vi "WriteExcel.vi"(8 "error in (no error)":errorcluster caption="错误输入（无错误）", 10 "Data":string[][](array[string]), 11 "Path":path=path "C:/Users/ct/Desktop/TestStep.xlsx") -> (0 "error out":errorcluster caption="错误输出")   [LabVIEW 2017]
uses:
  <vilib>/Utility/NIReport.llb/NI_report.lvclass
  <vilib>/Utility/NIReport.llb/Append Text Table to Report (wrap).vi
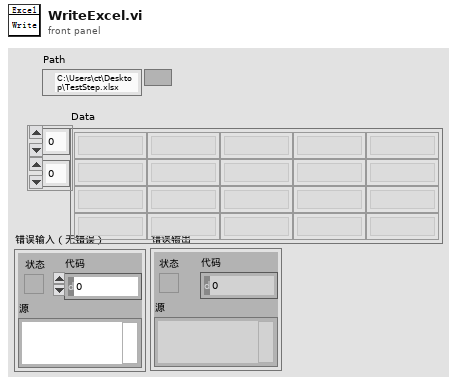
[diagram p1: front panel]
types:
  T1 = enum16{"Standard Report", "HTML", "Word", "Excel"}
  T2 = enum16{"maximized", "minimized", "normal", "no change"}
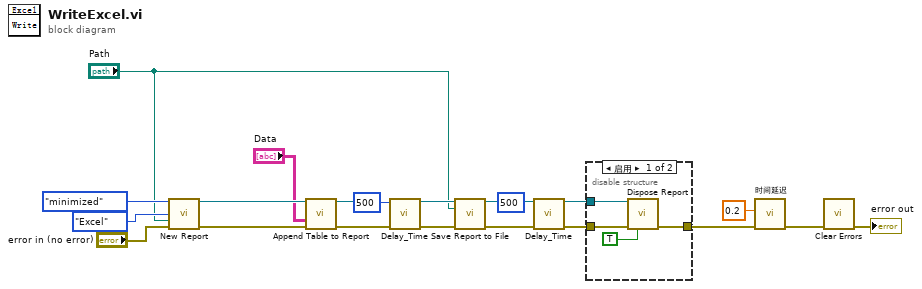
[diagram p0: block diagram]
diagram:
  n1 = call <vilib>:"New Report.vi"("window state (normal)"=T2."minimized", "report type"=T1."Excel", "template (empty)"="Path", "error in (no error)"="error in (no error)") -> ("report out"=w14:refnum<class "NI_report.lvclass">, "error out"=w13:errorcluster)  [unwired: 10 in]
  n2 = call-poly <vilib>:"Append Table to Report.vi"("report in"=w14, "text data"="Data", "error in (no error)"=w13) -> ("report out"=w8:refnum<class "NI_report.lvclass">, "error out"=w12:errorcluster)  [unwired: 9 in, 2 out]
  n3 = call "Delay_Time.vi"("error in (no error)"=w12, "Delay Time(ms)"=u32 500) -> ("error out"=w9:errorcluster)  [unwired: 9 in]
  n4 = call-dynamic "Save Report to File.vi"("report in"=w8, "report file path"="Path", "error in (no error)"=w9) -> ("report out"=w7:refnum<class "NI_report.lvclass">, "error out"=w5:errorcluster)  [unwired: 11 in]
  n5 = call "Delay_Time.vi"("error in (no error)"=w5, "Delay Time(ms)"=u32 500) -> ("error out"=w4:errorcluster)  [unwired: 9 in]
  n6 = disable-structure shown="启用" {
    disable-tunnel: [w22 _] -> w16
    disable-tunnel: w4 -> [w21 _]
    disable-tunnel: w7 -> [w20 _]
    frame Enabled {
      n7 = call-dynamic "Dispose Report.vi"("report in"=w20, "error in (no error)"=w21, "close report? (T)"=TRUE) -> ("error out"=w22:errorcluster)  [unwired: 12 in]
    }
    frame Disabled {
    }
  }
  n8 = call "时间延迟"("error in (no error)"=w16, "Delay Time (s)"=0.2) -> ("error out"=w2:errorcluster)  [unwired: 9 in]
  n9 = call <vilib>:"Clear Errors.vi"("error in (no error)"=w2) -> ("error out"=→"error out":errorcluster)  [unwired: 5 in, 1 out]
